vi "Asana_OAuth.vi"() -> ()   [LabVIEW 2016]
uses:
  <vilib>/httpClient/POSTBuffer.vi
  <vilib>/LVH/i3 JSON/JSON Parsing/Get Object Parameter Files/Get Object Parameter - String.vi
  <vilib>/httpClient/LabVIEWHTTPClient.lvlib
  <vilib>/LVH/i3 JSON/i3-json.lvlib
panel:
  in  "Hit when authorization is granted":bool
  out "new access_token authorization successful?":bool=TRUE
  out "new refresh_token authorization successful?":bool=TRUE
  in  "WebBrowser":refnum<k7>(container)
  out "refresh_token":string="0/e8deba2ebb8bd2d028329b434aa57d32"
  out "access_token":string="eyJ0eXAiOiJKV1QiLCJhbGciOiJIUzI1NiJ9.eyJhdXRob3JpemF0aW9uIjoxNTY3NDIwMDMxMjIyNywic2NvcGUiOiIiLCJpYXQiOjE1MTEyODIxOTksImV4cCI6MTUxMTI4NTc5OX0.3cbhR8T1RaZKz7Mp6LbDKKoba3BGVtEswHVRUv9TY6o"
  out "HTTP Returned Body":string="{\n  \"access_token\": \"eyJ0eXAiOiJKV1QiLCJhbGciOiJIUzI1NiJ9.eyJhdXRob3JpemF0aW9uIjoxNTY3NDIwMDMxMjIyNywic2NvcGUiOiIiLCJpYXQiOjE1MTEyODIxOTksImV4cCI6MTUxMTI4NTc5OX0.3cbhR8T1RaZKz7Mp6LbDKKoba3BGVtEswHVRUv9TY6o\",\n  \"token_type\": \"bearer\",\n  \"expires_in\": 3600,\n  \"data\": {\n    \"id\": 15435307170131,\n    \"name\": \"Yun-Yi Pai\",\n    \"email\": \"yun-yi.pai@pqi.org\"\n  }\n}"
  out "HTTP Returned Headers":string="HTTP/1.1 200 OK\r\nServer: nginx\r\nDate: Tue, 21 Nov 2017 16:36:39 GMT\r\nContent-Type: application/json; charset=UTF-8\r\nTransfer-Encoding: chunked\r\nConnection: keep-alive\r\nX-Frame-Options: SAMEORIGIN\r\nX-Content-Type-Options: nosniff\r\nX-XSS-Protection: 1; mode=block\r\nX-UA-Compatible: IE=edge,chrome=1\r\nContent-Security-Policy: report-uri /-/csp_report;script-src 'self' 'unsafe-eval' 'unsafe-inline' https://ssl.gstatic.com https://apis.google.com https://d3ki9tyy5l5ruj.cloudfront.net https://d1gwm4cf8hecp4.cloudfront.net https://d1a3usp4brejtz.cloudfront.net https://d3u0af8znnrzzj.cloudfront.net https://oauth.googleusercontent.com https://app.box.com https://platform.twitter.com https://connect.facebook.net https://platform.harvestapp.com https://www.google.com https://docs.google.com https://www.gstatic.com https://www.dropbox.com https://asana.recurly.com https://asanastage.recurly.com https://api.recurly.com https://js.recurly.com;child-src 'self' https://accounts.google.com https://content.googleapis.com https://www.google.com https://docs.google.com https://cdn.embedly.com https://fast.wistia.net https://www.dropbox.com https://platform.harvestapp.com https://www.googletagmanager.com https://asanaops.wufoo.com https://forms.asana.plus https://forms-server.asana.plus https://csv.asana.plus https://asana.com https://api.recurly.com https://pixel.asana.com https://d17ihzt85nhn2y.cloudfront.net\r\nCache-Control: no-store\r\nPragma: no-cache\r\nX-Asana-Content-String-Length: 359\r\nSet-Cookie: TooBusyRedirectCount=0\r\nX-Server-Name: prod-ws076.ec2\r\nX-Asana-Preferred-Release-Revision: 20171120_221241_867ba3e15db2221bfc1a505ff00d5822edf28beb\r\nX-Robots-Tag: none\r\nSet-Cookie: server=prod-ws076.ec2|WhRWG; path=/\r\nStrict-Transport-Security: max-age=31536000; includeSubDomains\r\nDatacenter-Time-End: 1511282199.319\r\nX-LoadBalancer: prod-lb008.ec2\r\n\r\n"
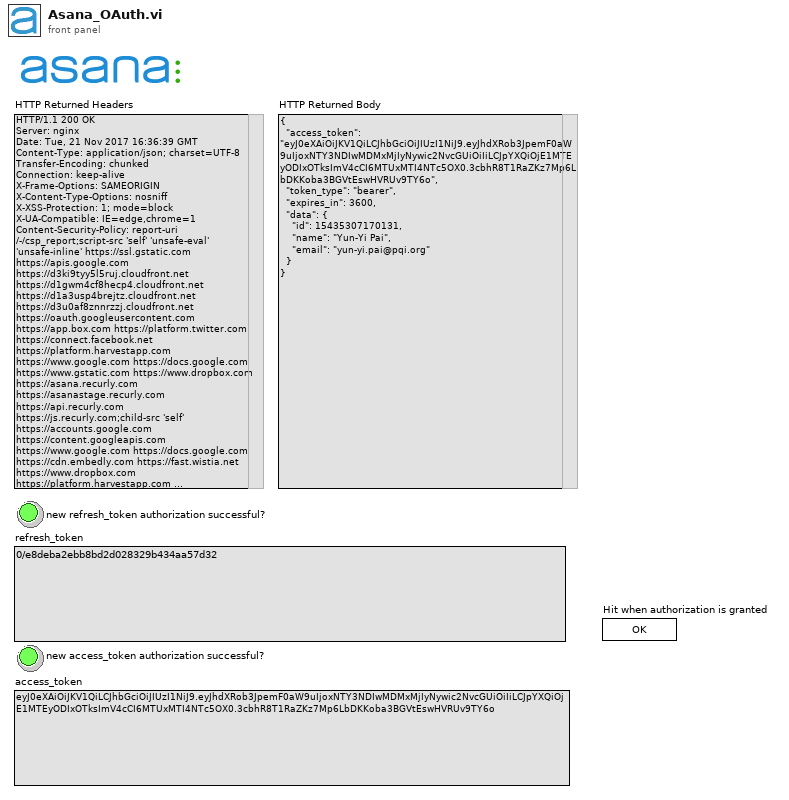
[diagram p1: front panel]
types:
  T1 = typedef "LabVIEWHTTPClient.lvlib/ClientHandle.ctl" = refnum<k1>
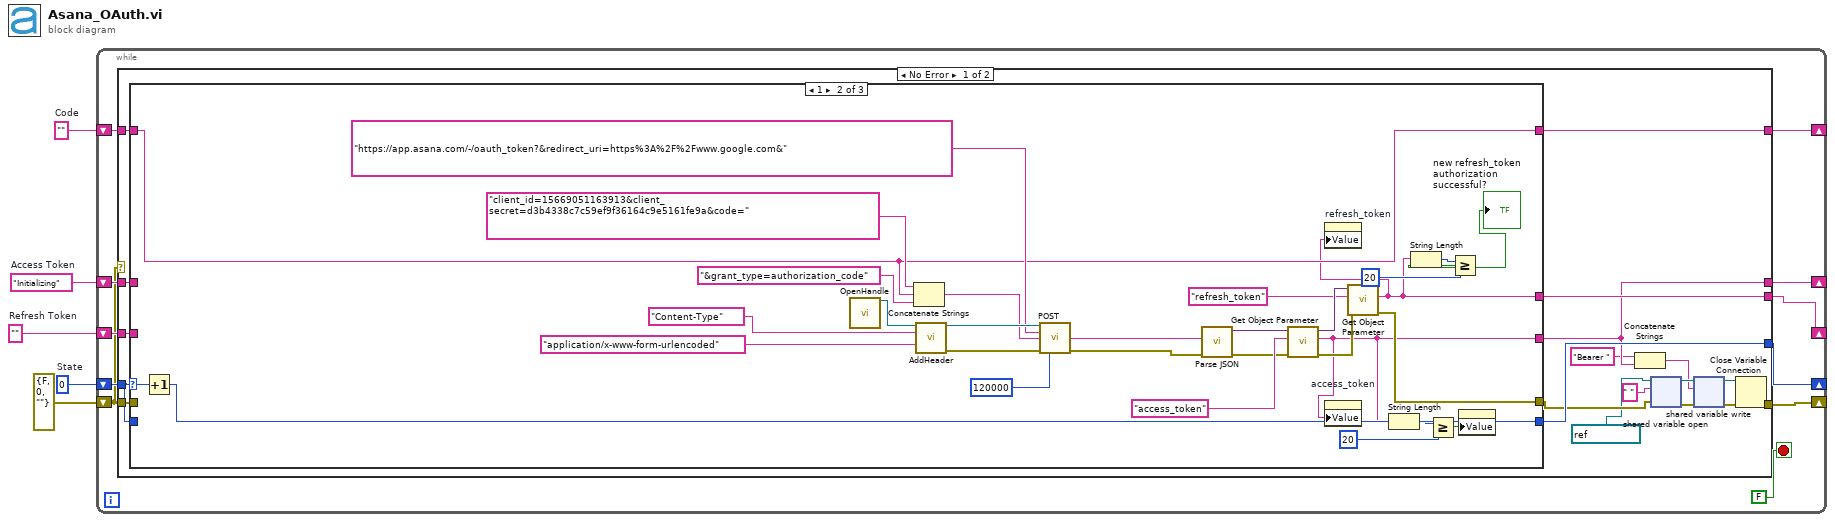
[diagram p0: block diagram]
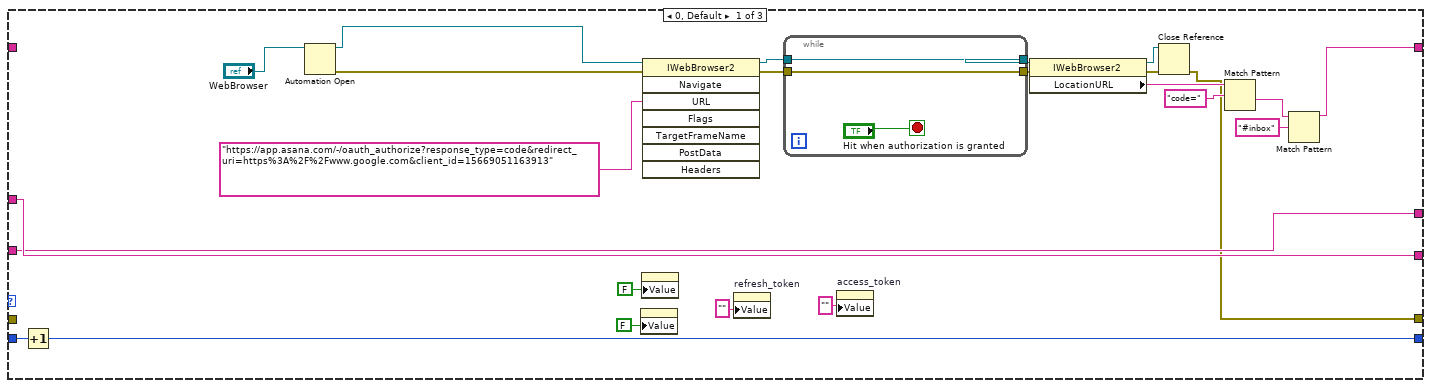
[diagram p2: hidden frame]
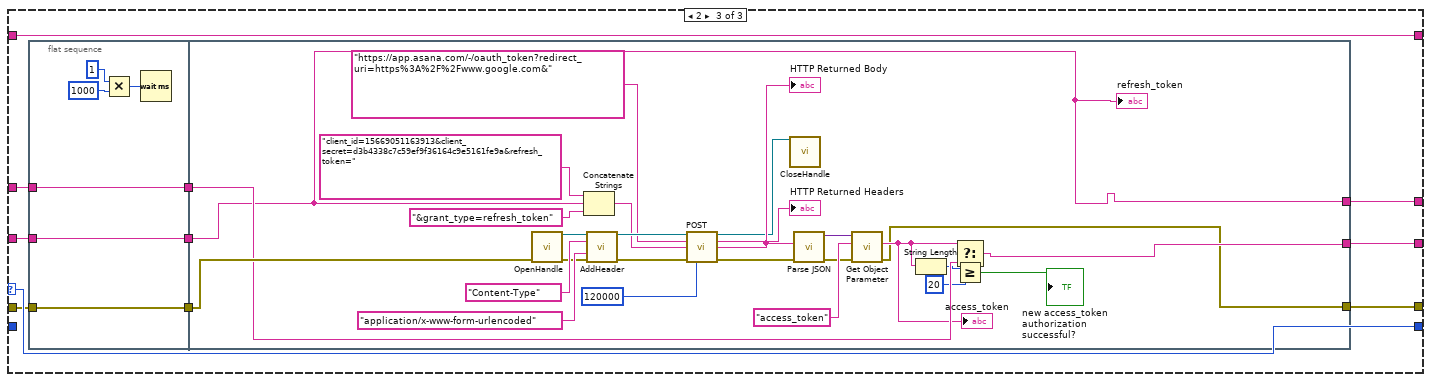
[diagram p3: hidden frame]
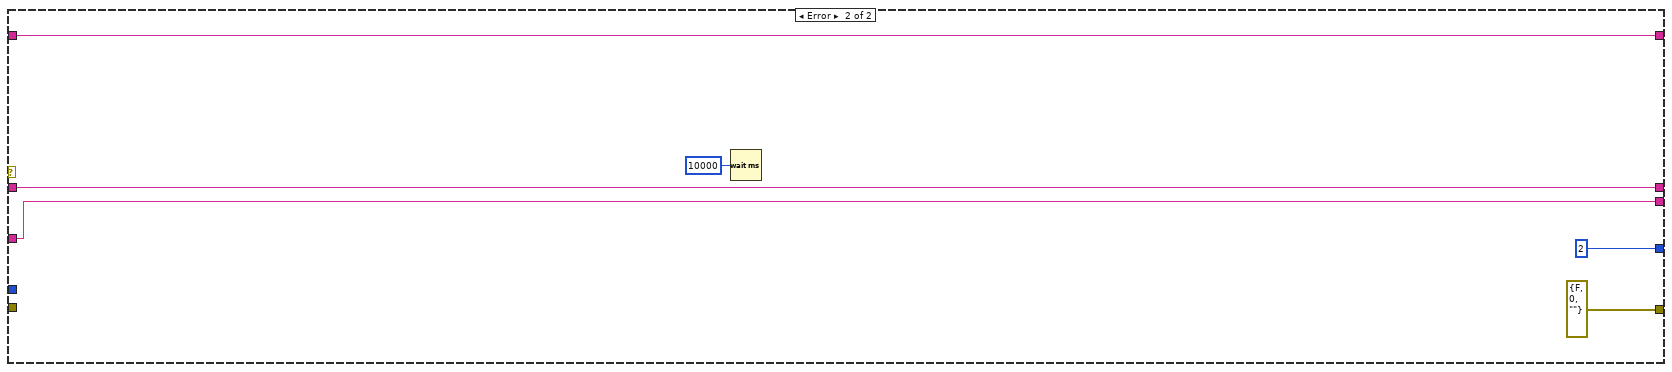
[diagram p4: hidden frame]
diagram:
  w2 = 0  # State
  w3 = ""  # Refresh Token
  w4 = "Initializing"  # Access Token
  w5 = ""  # Code
  n1 = while {
    shift-right: [w15] -> _
    shift-left: w2 -> [w10]
    shift-right: [w14] -> _
    shift-left: w5 -> [w13]
    shift-right: [w8] -> _
    shift-left: w4 -> [w9]
    shift-right: [w11] -> _
    shift-left: w3 -> [w12]
    shift-right: [w7] -> _
    shift-left: errorcluster {"status"=FALSE, "code"=0, "source"=""} ("error out") -> [w6]
    stop <- FALSE ("Stop Button 2") stop-if-true
    n2 = case shown="No Error" w6 {
      tunnel: [w35 2] -> w15
      tunnel: [w34 w137] -> w14
      tunnel: w13 -> [w33 w137]
      tunnel: w12 -> [w32 w138]
      tunnel: [w31 w138] -> w11
      tunnel: w10 -> [w30 _]
      tunnel: w9 -> [w24 w139]
      tunnel: [w23 w139] -> w8
      tunnel: [w20 errorcluster {"status"=FALSE, "code"=0, "source"=""} ("error out")] -> w7
      tunnel: w6 -> [w18 _]
      frame No Error {
        n3 = case shown="1" w30 {
          selector: w30 -> [_ w77 w103]
          tunnel: [w49 w64 w99] -> w31
          tunnel: [w50 w67 w100] -> w23
          tunnel: [w38 w75 w102] -> w34
          tunnel: [w48 w76 w103] -> w35
          tunnel: w33 -> [_ w75 w102]
          tunnel: w24 -> [w50 _ w94]
          tunnel: w32 -> [w49 _ w101]
          tunnel: w30 -> [w47 _ _]
          tunnel: [w46 w71 w93] -> w19
          tunnel: w18 -> [_ _ w97]
          frame 0, Default {
            n4 = Increment(x=w47) -> (x+1=w48:i32)
            n5 = Automation Open(Automation Refnum="WebBrowser") -> (Automation Refnum=w36:refnum<k7>, error out=w37:errorcluster)  [unwired: 3 in]
            n6 = property on="new access_token authorization successful?" class="Bool (strict)"("Value"=FALSE ("new access_token authorization successful?")) -> ()  [unwired: 2 in, 2 out]
            n7 = property on="new refresh_token authorization successful?" class="Bool (strict)"("Value"=FALSE ("new refresh_token authorization successful?")) -> ()  [unwired: 2 in, 2 out]
            n8 = invoke class="IWebBrowser2" method="Navigate"(reference=w36, error in=w37, "URL"="https://app.asana.com/-/oauth_authorize?response_type=code&redirect_uri=https%3A%2F%2Fwww.google.com&client_id=15669051163913") -> (reference out=w54:refnum<k7>, error out=w53:errorcluster)  [unwired: 5 in, 6 out]
            n9 = property on="refresh_token" class="Str"("Value"="") -> ()  [unwired: 2 in, 2 out]
            n10 = while {
              tunnel: [w62] -> w52
              tunnel: w54 -> [w62]
              tunnel: [w61] -> w51
              tunnel: w53 -> [w61]
              stop <- "Hit when authorization is granted" stop-if-true
            }
            n11 = property on="access_token" class="Str"("Value"="") -> ()  [unwired: 2 in, 2 out]
            n12 = property class="IWebBrowser2"(reference=w52, error in=w51) -> (reference out=w59:refnum<k7>, error out=w58:errorcluster, "LocationURL"=w56:string)
            n13 = Close Reference(reference=w59, error in (no error)=w58) -> (error out=w46:errorcluster)
            n14 = Match Pattern(string=w56, regular expression="code=") -> (after substring=w39:string)  [unwired: 1 in, 3 out]
            n15 = Match Pattern(string=w39, regular expression="#inbox") -> (before substring=w38:string)  [unwired: 1 in, 3 out]
          }
          frame 1 {
            n16 = Increment(x=w77) -> (x+1=w76:i32)
            n17 = call <vilib>:"OpenHandle.vi"() -> ("client handle out"=w87:T1)  [unwired: 14 in, 1 out]
            n18 = Concatenate Strings("client_id=15669051163913&client_secret=d3b4338c7c59ef9f36164c9e5161fe9a&code=" ("text"), w75, "&grant_type=authorization_code" ("string")) -> (w86:string)
            n19 = call <vilib>:"AddHeader.vi"("client handle"=w87, "header"="Content-Type", "value"="application/x-www-form-urlencoded") -> ("client handle out"=w92:T1, "error out"=w83:errorcluster)  [unwired: 11 in]
            n20 = call-poly <vilib>:"POST.vi"("client handle"=w92, "url"="https://app.asana.com/-/oauth_token?&redirect_uri=https%3A%2F%2Fwww.google.com&", "buffer"=w86, "error in (no error)"=w83, "timeout (10000)"=120000) -> ("body"=w82:string, "error out"=w74:errorcluster)  [unwired: 7 in, 2 out]
            n21 = call <vilib>:"Parse JSON.vi"("error in (no error)"=w74, "JSON String"=w82) -> ("error out"=w73:errorcluster, "JSON Tree"=w81:variant)  [unwired: 6 in, 2 out]
            n22 = call-poly <vilib>:"Get Object Parameter.vi"("error in (no error)"=w73, "Parameter Name"="access_token", "JSON Tree In (JSON Object)"=w81) -> ("error out"=w72:errorcluster, "String Value"=w67:string, "JSON Tree Out Passthrough"=w80:variant)  [unwired: 5 in, 1 out]
            n23 = property on="access_token" class="Str"("Value"=w67) -> ()  [unwired: 2 in, 2 out]
            n24 = call-poly <vilib>:"Get Object Parameter.vi"("error in (no error)"=w72, "Parameter Name"="refresh_token", "JSON Tree In (JSON Object)"=w80) -> ("error out"=w71:errorcluster, "String Value"=w64:string)  [unwired: 5 in, 2 out]
            n25 = property on="refresh_token" class="Str"("Value"=w64) -> ()  [unwired: 2 in, 2 out]
            n26 = String Length(string=w67) -> (length=w68:i32)
            n27 = String Length(string=w64) -> (length=w65:i32)
            n28 = Greater Or Equal?(x=w68, y=20) -> (x >= y?=w70:bool)
            n29 = Greater Or Equal?(x=w65, y=20) -> (x >= y?=→"new refresh_token authorization successful?":bool)
            n30 = property on="new access_token authorization successful?" class="Bool (strict)"("Value"=w70) -> ()  [unwired: 2 in, 2 out]
          }
          frame 2 {
            n31 = flat-sequence {
              tunnel: w101 -> [w109]
              tunnel: [w109] -> w98
              tunnel: w97 -> [w105]
              tunnel: [w105] -> w96
              tunnel: [w104] -> w95
              tunnel: w94 -> [w104]
              tunnel: [w117] -> w100
              tunnel: [w111] -> w99
              tunnel: w98 -> [w111]
              tunnel: w96 -> [w120]
              tunnel: w95 -> [w116]
              tunnel: [w110] -> w93
              frame #0 {
                n32 = Multiply(x=u32 1 ("milliseconds to wait"), y=u32 1000) -> (x*y=w107:u32)
                n33 = Wait (ms)(milliseconds to wait=w107) -> ()  [unwired: 1 out]
              }
              frame #1 {
                n34 = call <vilib>:"OpenHandle.vi"("error in (no error)"=w120) -> ("client handle out"=w128:T1, "error out"=w119:errorcluster)  [unwired: 13 in]
                n35 = Concatenate Strings("client_id=15669051163913&client_secret=d3b4338c7c59ef9f36164c9e5161fe9a&refresh_token=" ("text"), w111, "&grant_type=refresh_token" ("string")) -> (w127:string)
                n36 = call <vilib>:"AddHeader.vi"("client handle"=w128, "header"="Content-Type", "value"="application/x-www-form-urlencoded", "error in (no error)"=w119) -> ("client handle out"=w133:T1, "error out"=w123:errorcluster)  [unwired: 10 in]
                n37 = call-poly <vilib>:"POST.vi"("client handle"=w133, "url"="https://app.asana.com/-/oauth_token?redirect_uri=https%3A%2F%2Fwww.google.com&", "buffer"=w127, "error in (no error)"=w123, "timeout (10000)"=120000) -> ("client handle out"=w121:T1, "headers"=→"HTTP Returned Headers":string, "body"=w126:string, "error out"=w122:errorcluster)  [unwired: 7 in]
                "HTTP Returned Body" <- w126
                n38 = call <vilib>:"CloseHandle.vi"("client handle"=w121) -> ()  [unwired: 14 in, 1 out]
                n39 = call <vilib>:"Parse JSON.vi"("error in (no error)"=w122, "JSON String"=w126) -> ("error out"=w118:errorcluster, "JSON Tree"=w125:variant)  [unwired: 6 in, 2 out]
                n40 = call-poly <vilib>:"Get Object Parameter.vi"("error in (no error)"=w118, "Parameter Name"="access_token", "JSON Tree In (JSON Object)"=w125) -> ("error out"=w110:errorcluster, "String Value"=w113:string)  [unwired: 5 in, 2 out]
                "access_token" <- w113
                n41 = String Length(string=w113) -> (length=w115:i32)
                n42 = Greater Or Equal?(x=w115, y=20) -> (x >= y?=w112:bool)
                "new access_token authorization successful?" <- w112
                n43 = Select(t=w113, s=w112, f=w116) -> (s? t:f=w117:string)
                "refresh_token" <- w111
              }
            }
          }
        }
        n44 = Concatenate Strings("Bearer " ("string"), w23) -> (w22:string)
        n45 = shared-variable-open(refnum<k21> "ni.var.psp://housesoftheholy/OneNote API HTTP/Asana Access Token 15669051163913" ("shared variable refnum in"), w19, " " ("string")) -> (w28:refnum<k21>, w27:errorcluster)  [unwired: 1 in]
        n46 = shared-variable-write(w28, w27, w22) -> (w29:refnum<k21>, w26:errorcluster)
        n47 = Close Variable Connection(8:w26, 11:w29) -> (0:w20:errorcluster)
      }
      frame Error {
        n48 = Wait (ms)(milliseconds to wait=u32 10000) -> ()  [unwired: 1 out]
      }
    }
  }
